vi "LFA_AcquireWithAutosave.vi"(8 "error in (no error)":errorcluster, 11 "LightField Automation in":refnum<class "LightField Automation.lvclass">) -> (0 "error out":errorcluster, 2 "Data":T1(array[cluster]), 3 "LightField Automation out":refnum<class "LightField Automation.lvclass">)   [LabVIEW 2018, in "LightField Automation.lvclass"]
uses:
  LightField Automation.lvclass
  LightField Automation.lvclass/LightField Automation.ctl
  C:/Program Files/Princeton Instruments/LightField/AddInViews/PrincetonInstruments.LightFieldViewV3.dll
  Program Files/Princeton Instruments/LightField/AddInViews/PrincetonInstruments.LightFieldViewV3.dll
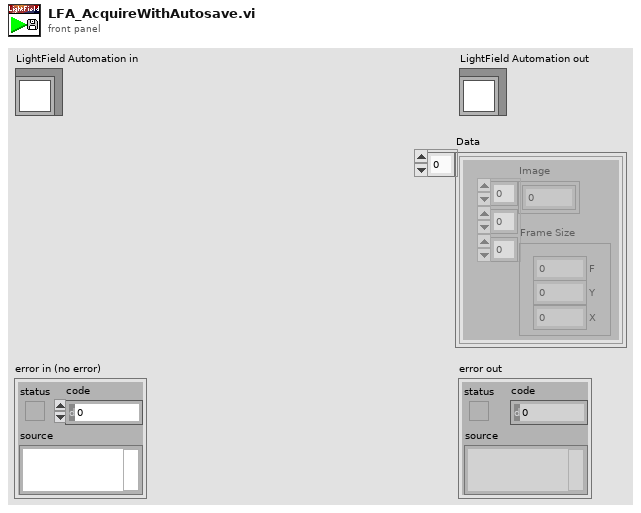
[diagram p1: front panel]
types:
  T1 = cluster{"Image":dbl[][][], "Frame Size":cluster{"F":i32, "Y":i32, "X":i32}}[]
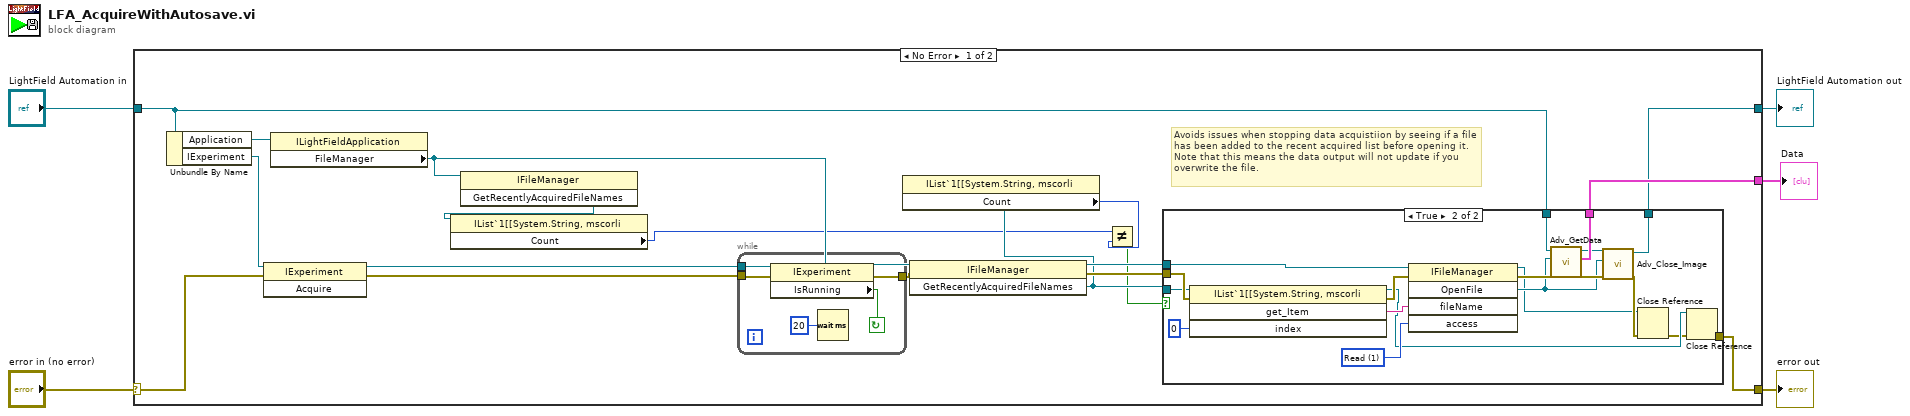
[diagram p0: block diagram]
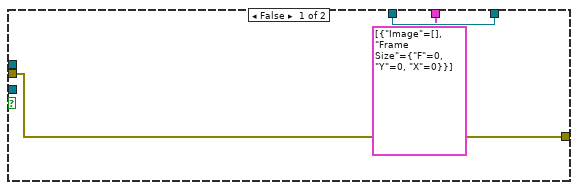
[diagram p2: hidden frame]
diagram:
  n1 = case shown="No Error" "error in (no error)" {
    selector: "error in (no error)" -> [w23 w52]
    tunnel: [w13 w52] -> w4
    tunnel: [w12 w51] -> w2
    tunnel: "LightField Automation in" -> [w19 w51]
    tunnel: [w18 _] -> w1
    frame No Error {
      # "Avoids issues when stopping data acquistiion by seeing if a file has been added to the recent acquired list before opening it. Note that this means the data output will not update if you overwrite the file."
      n2 = Unbundle By Name(w19) -> ("Application"=w17:refnum<k24>, "IExperiment"=w20:refnum<k24>)
      n3 = invoke class="IExperiment" method="Acquire"(reference=w20, error in=w23) -> (reference out=w21:refnum<k24>, error out=w22:errorcluster)  [unwired: 1 in, 1 out]
      n4 = property class="ILightFieldApplication"(reference=w17) -> ("FileManager"=w10:refnum<k24>)  [unwired: 1 in, 2 out]
      n5 = invoke class="IFileManager" method="GetRecentlyAcquiredFileNames"(reference=w10) -> ("GetRecentlyAcquiredFileNames"=w9:refnum<k24>)  [unwired: 2 in, 2 out]
      n6 = property class="IList`1[[System.String, mscorli"(reference=w9) -> ("Count"=w8:i32)  [unwired: 1 in, 2 out]
      n7 = while {
        tunnel: w22 -> [w48]
        tunnel: [w47] -> w16
        tunnel: w21 -> [w46]
        stop <- w50 continue-if-true
        n8 = property class="IExperiment"(reference=w46, error in=w48) -> (error out=w47:errorcluster, "IsRunning"=w50:bool)  [unwired: 1 out]
        n9 = Wait (ms)(milliseconds to wait=u32 20) -> ()  [unwired: 1 out]
      }
      n10 = invoke class="IFileManager" method="GetRecentlyAcquiredFileNames"(reference=w10, error in=w16) -> (reference out=w14:refnum<k24>, error out=w15:errorcluster, "GetRecentlyAcquiredFileNames"=w11:refnum<k24>)  [unwired: 1 in]
      n11 = property class="IList`1[[System.String, mscorli"(reference=w11) -> ("Count"=w7:i32)  [unwired: 1 in, 2 out]
      n12 = Not Equal?(x=w8, y=w7) -> (x != y?=w6:bool)
      n13 = case shown="True" w6 {
        tunnel: w19 -> [w25 w45]
        tunnel: [T1 [{"Image"=[], "Frame Size"={"F"=0, "Y"=0, "X"=0}}] ("Data") w44] -> w18
        tunnel: w15 -> [w26 w43]
        tunnel: w14 -> [_ w40]
        tunnel: [w26 w36] -> w13
        tunnel: [w25 w32] -> w12
        tunnel: w11 -> [_ w27]
        frame False {
        }
        frame True {
          w38 = 1 items=["Read"=1, "Write"=2, "ReadWrite"=3] ("access")
          n14 = invoke class="IList`1[[System.String, mscorli" method="get_Item"(reference=w27, error in=w43, "index"=0) -> (reference out=w35:refnum<k24>, error out=w41:errorcluster, "get_Item"=w39:string)  [unwired: 1 in, 1 out]
          n15 = invoke class="IFileManager" method="OpenFile"(reference=w40, error in=w41, "fileName"=w39, "access"=w38) -> (reference out=w28:refnum<k24>, error out=w37:errorcluster, "OpenFile"=w29:refnum<k24>)  [unwired: 1 in, 2 out]
          n16 = call "Adv_GetData.vi"("error in (no error)"=w37, "IImageDataSet"=w29, "LightField Automation in"=w45) -> ("error out"=w34:errorcluster, "Data"=w44:T1, "LightField Automation out"=w33:refnum<class "LightField Automation.lvclass">)  [unwired: 6 in]
          n17 = call "Adv_Close_Image.vi"("error in (no error)"=w34, "ImageDataSet"=w29, "LightField Automation in"=w33) -> ("error out"=w30:errorcluster, "LightField Automation out"=w32:refnum<class "LightField Automation.lvclass">)  [unwired: 7 in]
          n18 = Close Reference(reference=w28, error in (no error)=w30) -> (error out=w31:errorcluster)
          n19 = Close Reference(reference=w35, error in (no error)=w31) -> (error out=w36:errorcluster)
        }
      }
    }
    frame Error {
    }
  }
  "error out" <- w4
  "LightField Automation out" <- w2
  "Data" <- w1
